vi "计算直流分量子程序.vi"(1 "波形":waveform(dbl)) -> (0 "直流分量":dbl)   [LabVIEW 2017]
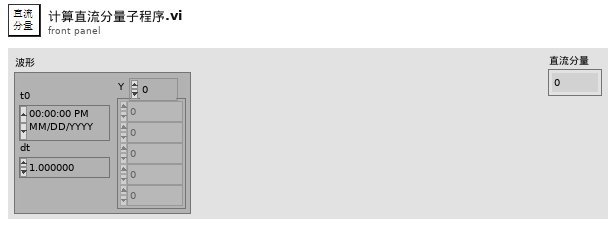
[diagram p1: front panel]
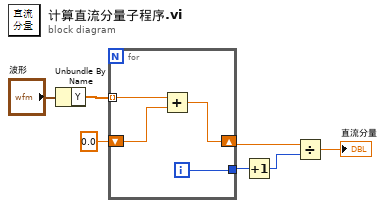
[diagram p0: block diagram]
diagram:
  n1 = Unbundle By Name("波形") -> ("Y"=w6:dbl[])
  n2 = for {
    tunnel: w6 -> [w11] mode=indexing
    shift-right: [w9] -> w3
    shift-left: 0.0 -> [w10]
    tunnel: [w8] -> w4
    i -> [w8]
    n3 = Add(x=w11, y=w10) -> (x+y=w9:dbl)
  }
  n4 = Increment(x=w4) -> (x+1=w2:i32)
  n5 = Divide(x=w3, y=w2) -> (x/y=→"直流分量":dbl)
